vi "OMV_Txbuffer.vi"(8 "error in (no error)":errorcluster, 11 "Python":T1) -> (0 "error out":errorcluster, 2 "Data":dbl[](array[numeric]), 3 "Python":T1)   [LabVIEW 2020]
uses:
  PythonCtrl.ctl
  _subs/Processors.ctl
panel:
  out "Tx Buffer":string
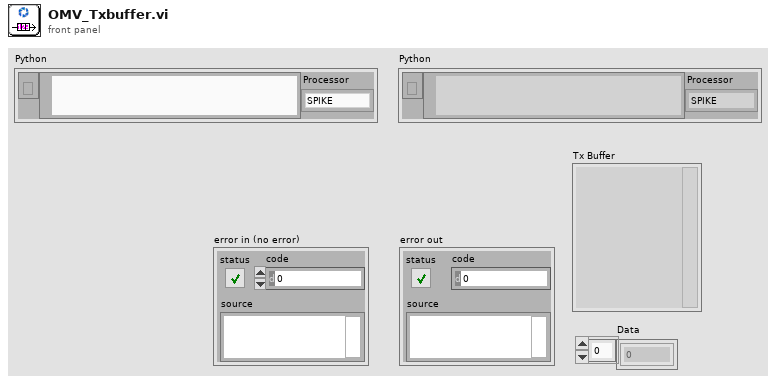
[diagram p1: front panel]
types:
  T1 = typedef "PythonCtrl.ctl" = cluster{"session":refnum<k35>, "PyPath":path, "Processor":T2}
  T2 = typedef "Processors.ctl" = enum16{"SPIKE", "Pi", "Pi_ssh", "OpenMV"}
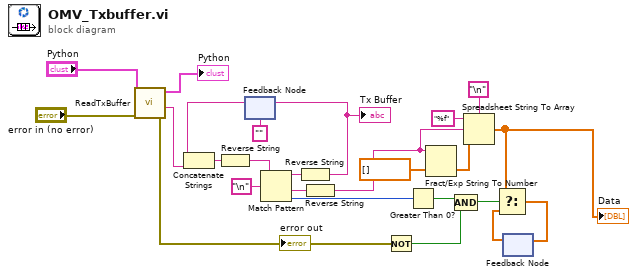
[diagram p0: block diagram]
diagram:
  n1 = call "ReadTxBuffer.vi"("error in"="error in (no error)", "Python"="Python") -> ("error out"=w17:errorcluster, "Tx Buffer"=w15:string, "Python"=→"Python":T1)  [unwired: 6 in, 1 out]
  "error out" <- w17
  n2 = feedback #1("") -> (w12:string)
  n3 = Concatenate Strings(w12, w15) -> (w13:string)
  n4 = Reverse String(1:w13) -> (0:w6:string)
  n5 = Match Pattern(string=w6, regular expression="\n") -> (before substring=w5:string, after substring=w4:string, offset past match=w14:i32)  [unwired: 1 in, 1 out]
  n6 = Reverse String(1:w5) -> (0:w3:string)
  "Tx Buffer" <- w3
  n7 = feedback-in #1(w3) -> ()
  n8 = Reverse String(1:w4) -> (0:w2:string)
  n9 = Not(x=w17) -> (.not. x?=w16:bool)
  n10 = Greater Than 0?(x=w14) -> (x > 0?=w20:bool)
  n11 = Fract/Exp String To Number(string=w2) -> ()  [unwired: 3 in, 2 out]
  n12 = Compound Arithmetic op=AND(w20, w16) -> (w19:bool)
  n13 = Spreadsheet String To Array(delimiter (Tab)="\n", format string="%f", spreadsheet string=w2, array type (2D Dbl)=dbl[] [] ("Data")) -> (array=w1:dbl[])
  "Data" <- w1
  n14 = feedback #2() -> (w21:dbl[])  [unwired: 1 in]
  n15 = Select(t=w1, s=w19, f=w21) -> (s? t:f=w7:dbl[])
  n16 = feedback-in #2(w7) -> ()
